vi "Stop Panel.vi"(6 "Panel Host":refnum<vi>, 8 "error in (no error)":errorcluster, 9 "Panel":enum16{"UI Setting Panel", "Output Panel"}(ring), 10 "Panel VI in":refnum<vi>, 11 "UIStep in":refnum<class "UIStep.lvclass">) -> (0 "error out":errorcluster, 3 "UIStep out":refnum<class "UIStep.lvclass">)   [LabVIEW 2015, in "UIStep.lvclass"]
uses:
  UIStep.lvclass
  Step.lvclass
  Project.lvclass
  Editor/Editor.lvclass
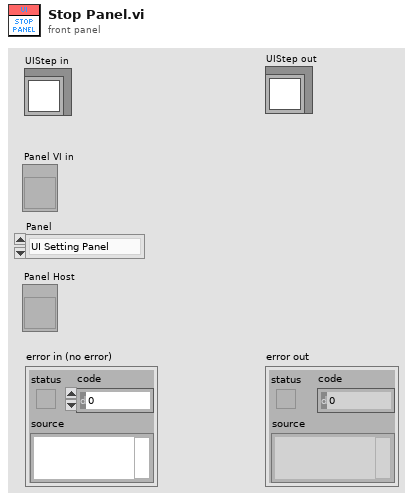
[diagram p1: front panel]
types:
  T1 = typedef "Step.lvclass/STEP_OUTPUT.ctl" = cluster{"Label":string, "Name":string, "Data Type":T2, "Check Type":T3, "String Limit":string, "Lower Limit":dbl, "Upper Limit":dbl, "Boolean Limit":bool, "Ignore Case":bool, "Variable Name 1":string, "Limit Value Type 1":T4, "Variable Name 2":string, "Limit Value Type 2":T4}
  T2 = typedef "Step.lvclass/OUTPUT_DATA_TYPE.ctl" = enum16{"Boolean", "String", "Numeric", "Other"}
  T3 = typedef "Step.lvclass/OUTPUT_CHECK_TYPE.ctl" = enum16{"INVALID", "DO_NOT_CHECK", "RECORD", "VARIABLE", "EQUAL", "NOT_EQUAL", "STR_CONTAINS", "STR_START_WITH", "STR_END_WITH", "STR_REGEX_MATCH", "NUM_GT", "NUM_LT", "NUM_GE", "NUM_LE", "NUM_RANGE", "NUM_RANGE_BDY"}
  T4 = typedef "Step.lvclass/OUTPUT_VALUE_TYPE.ctl" = enum16{"Constant", "Variable"}
  T5 = cluster{"Font":string, "Size":dbl, "Justification":u16, "TextColor":u32, "BGColor":u32, "Bold":bool}
  T6 = cluster{"Button1":cluster{"Label":string, "Size":dbl, "TextColor":u32, "BGColor":u32, "Bold":bool}, "Button2":cluster{"Label":string, "Size":dbl, "TextColor":u32, "BGColor":u32, "Bold":bool}}
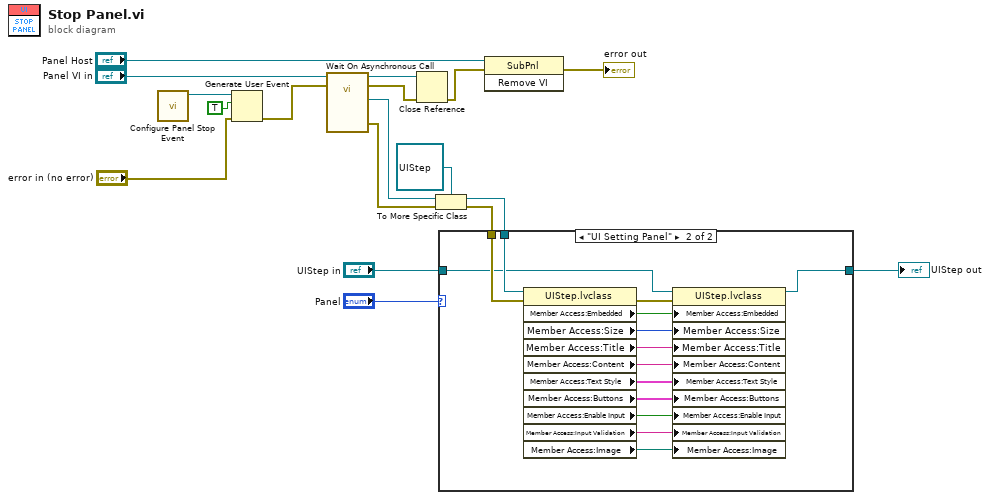
[diagram p0: block diagram]
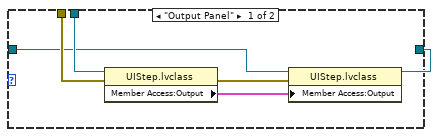
[diagram p2: hidden frame]
diagram:
  n1 = call "Configure Panel Stop Event.vi"() -> ("Panel Stop event"=w14:refnum<user-event>)  [unwired: 11 in]
  n2 = Generate User Event(user event=w14, event data cluster=TRUE, error in="error in (no error)") -> (error out=w12:errorcluster)  [unwired: 1 in, 1 out]
  n3 = call-by-ref "Wait On Asynchronous Call"(reference="Panel VI in", error in=w12) -> (reference out=w18:refnum<vi>, error out=w17:errorcluster, 0:"error out"=w8:errorcluster, "Step out"=w7:refnum<class "Step.lvclass">)  [unwired: 10 in]
  n4 = Close Reference(reference=w18, error in (no error)=w17) -> (error out=w11:errorcluster)
  n5 = To More Specific Class(target class=refnum<class "UIStep.lvclass"> refnum ("UIStep in"), reference=w7, error in=w8) -> (specific class reference=w5:refnum<class "UIStep.lvclass">, error out=w6:errorcluster)
  n6 = case shown="\"UI Setting Panel\"" "Panel" {
    tunnel: w5 -> [w24 w38]
    tunnel: w6 -> [w23 w37]
    tunnel: "UIStep in" -> [w22 w36]
    tunnel: [w20 w35] -> w3
    frame "Output Panel" {
      n7 = property class="UIStep.lvclass"(reference=w24, error in=w23) -> (error out=w19:errorcluster, "Member Access:Output"=w21:T1[])  [unwired: 1 out]
      n8 = property class="UIStep.lvclass"(reference=w22, error in=w19, "Member Access:Output"=w21) -> (reference out=w20:refnum<class "UIStep.lvclass">)  [unwired: 1 out]
    }
    frame "UI Setting Panel" {
      n9 = property class="UIStep.lvclass"(reference=w38, error in=w37) -> (error out=w34:errorcluster, "Member Access:Embedded"=w33:bool, "Member Access:Size"=w32:enum16{"Small", "Middle", "Big"}, "Member Access:Title"=w31:string, "Member Access:Content"=w30:string, "Member Access:Text Style"=w29:T5, "Member Access:Buttons"=w28:T6, "Member Access:Enable Input"=w27:bool, "Member Access:Input Validation"=w26:string, "Member Access:Image"=w25:path)  [unwired: 1 out]
      n10 = property class="UIStep.lvclass"(reference=w36, error in=w34, "Member Access:Embedded"=w33, "Member Access:Size"=w32, "Member Access:Title"=w31, "Member Access:Content"=w30, "Member Access:Text Style"=w29, "Member Access:Buttons"=w28, "Member Access:Enable Input"=w27, "Member Access:Input Validation"=w26, "Member Access:Image"=w25) -> (reference out=w35:refnum<class "UIStep.lvclass">)  [unwired: 1 out]
    }
  }
  "UIStep out" <- w3
  n11 = invoke class="SubPnl" method="Remove VI"(reference="Panel Host", error in=w11) -> (error out=→"error out":errorcluster)  [unwired: 1 in, 2 out]
